vi "Real Matrix Logarithm.vi"(2 "logarithm option":T1 items=["General", "Real"], 3 "Input Matrix":T3) -> (0 "error":i32, 1 "Matrix Logarithm":T2)   [LabVIEW 2020, in "NI_AALBase.lvlib"]
doc: "Computes the natural logarithm of a square <B>Input Matrix</B>. Wire data to the <B>Input Matrix</B> input to determine the polymorphic instance to use or manually select the instance."
uses:
  <vilib>/Analysis/NI_AALBase.lvlib
  <vilib>/Analysis/Matrix/Datatypes/RealMatrix.ctl
  <vilib>/Analysis/Matrix/Datatypes/ComplexMatrix.ctl
  <vilib>/Analysis/7linalg.llb/Matrix Logarithm Option.ctl
  <vilib>/Analysis/Matrix/Numeric/Complex/Cartesian To Complex - RM,R.vi
  <resource>/lvanlys.dll
  <vilib>/Analysis/Matrix/NI_Matrix.lvlib
panel:
  # "Real Matrix Logarithm"
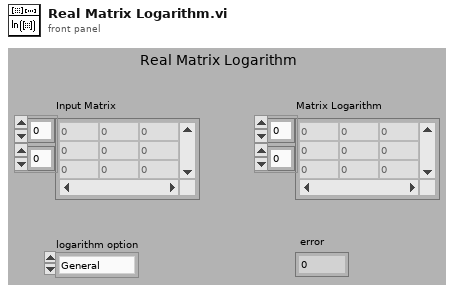
[diagram p1: front panel]
types:
  T1 = typedef "NI_AALBase.lvlib/Matrix Logarithm Option.ctl" = u16
  T2 = typedef "NI_Matrix.lvlib/ComplexMatrix.ctl" = cdb[][]
  T3 = typedef "NI_Matrix.lvlib/RealMatrix.ctl" = dbl[][]
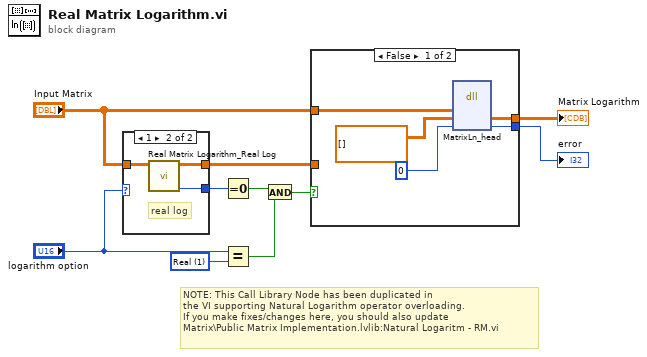
[diagram p0: block diagram]
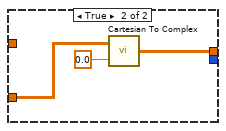
[diagram p2: hidden frame]
diagram:
  w1 = T1 1 items=["General", "Real"] ("y")
  # "NOTE: This Call Library Node has been duplicated in\nthe VI supporting Natural Logarithm operator overloading.\nIf you make fixes/changes here, you should also update\nMatrix\\Public Matrix Implementation.lvlib:Natural Logaritm - RM.vi"
  n1 = case shown="1" "logarithm option" {
    tunnel: "Input Matrix" -> [_ w13]
    tunnel: [_ w12] -> w4
    tunnel: [_ w11] -> w7
    frame 0, Default {
    }
    frame 1 {
      # "real log"
      n2 = call <vilib>:"Real Matrix Logarithm_Real Log.vi"("Input Matrix"=w13) -> ("error"=w11:i32, "Matrix Logarithm"=w12:T3)  [unwired: 9 in]
    }
  }
  n3 = Equal To 0?(x=w7) -> (x = 0?=w6:bool)
  n4 = Equal?(x="logarithm option", y=w1) -> (x = y?=w2:bool)
  n5 = And(x=w6, y=w2) -> (x .and. y?=w5:bool)
  n6 = case shown="False" w5 {
    tunnel: "Input Matrix" -> [w18 _]
    tunnel: [w17 _] -> w10
    tunnel: [w16 w19] -> w9
    tunnel: w4 -> [_ w21]
    frame False {
      n7 = dll-call lib="e:/builds/penguin/labview/branches/2020/dev/dist/resource/lvanlys.*" fn="MatrixLn_head"("Input Matrix"=w18, T2 [] ("Matrix Logarithm"), 0) -> (w16:T2, w17:i32)  [unwired: 5 in, 2 out]
    }
    frame True {
      n8 = call-poly <vilib>:"Cartesian To Complex.vi"("Real Scalar k"=0.0, "Real Matrix R"=w21) -> ("R + ki"=w19:T2)
    }
  }
  "Matrix Logarithm" <- w9
  "error" <- w10
